vi "Collect Method Results.vi"(10 "Test Method Result":T1, 11 "Report Generator In":refnum<class "Result Collector.lvclass">) -> (3 "Report Generator Out":refnum<class "Result Collector.lvclass">)   [LabVIEW 2020, in "Result Collector.lvclass"]
uses:
  Result Collector.lvclass
  Result Types/Assertion Result/Public/TypeDefs/Status.ctl
  Result Types/Assertion Result/Assertion Result.lvlib
  Result Types/Assertion Result/Public/TypeDefs/Assertion Type.ctl
  Result Types/Assertion Result/Assertion Result.ctl
  Result Types/Method Result/Method Result.ctl
  Result Types/Method Result/Method Result.lvlib
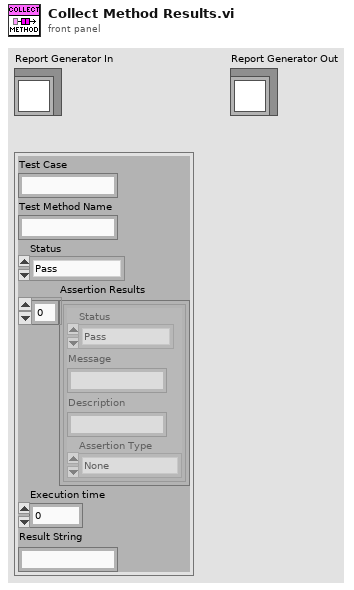
[diagram p1: front panel]
types:
  T1 = typedef "Method Result.lvlib/Method Result.ctl" = cluster{"Test Case":string, "Test Method Name":string, "Status":T2, "Assertion Results":T3[], "Execution time":dbl, "Result String":string}
  T2 = typedef "Assertion Result.lvlib/Status.ctl" = enum16{"Pass", "Fail", "Error", "Skipped", "Setup Error", "Broken", "Teardown Error"}
  T3 = typedef "Assertion Result.lvlib/Assertion Result.ctl" = cluster{"Status":T2, "Message":string, "Description":string, "Assertion Type":T4}
  T4 = typedef "Assertion Result.lvlib/Assertion Type.ctl" = enum16{"None", "Pass", "Fail", "Skip", "Pass if Equal", "Fail if Equal", "Pass if Error", "Fail if Error", "Pass if", "Fail if"}
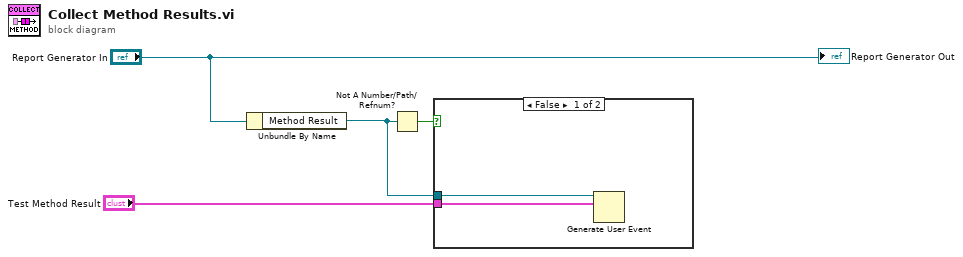
[diagram p0: block diagram]
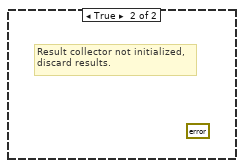
[diagram p2: hidden frame]
diagram:
  n1 = Unbundle By Name("Report Generator In") -> ("Method Result"=w1:refnum<user-event>)
  n2 = Not A Number/Path/Refnum?(number/path/refnum=w1) -> (NaN/Path/Refnum?=w2:bool)
  n3 = case shown="False" w2 {
    tunnel: "Test Method Result" -> [w6 _]
    tunnel: w1 -> [w5 _]
    frame False {
      n4 = Generate User Event(user event=w5, event data cluster=w6) -> ()  [unwired: 2 in, 2 out]
    }
    frame True {
      (unwired) errorcluster {"status"=FALSE, "code"=0, "source"=""} ("error out")
      # "Result collector not initialized,\ndiscard results."
    }
  }
  "Report Generator Out" <- "Report Generator In"
